vi "setUp.vi"(8 "error in (no error)":errorcluster, 11 "reference in":refnum<class "Import Export Test.lvclass">) -> (0 "error out":errorcluster, 3 "reference out":refnum<class "Import Export Test.lvclass">)   [LabVIEW 2019, in "Import Export Test.lvclass"]
doc: "setUp runs prior to the test method during test execution. Use this method to initialize any object data required by your tests."
uses:
  Import Export Test.lvclass
  C:/Program Files (x86)/National Instruments/LabVIEW 2019/vi.lib/addons/_JKI Toolkits/VI Tester/TestCase.llb/TestCase.lvclass
  NationalInstruments.VeriStand.SystemDefinitionAPI
  Import Export Test.lvclass/Import Export Test.ctl
  <userlib>/_OpenG.lib/file/file.llb/Append Path to Root if Relative - Scalar__ogtk.vi
  <vilib>/addons/_JKI Toolkits/VI Tester/TestCase.llb/TestCase.lvclass
  niveristand-custom-device-testing-tools/VeriStandTestUtilities/VeriStandTestUtilities.lvlib
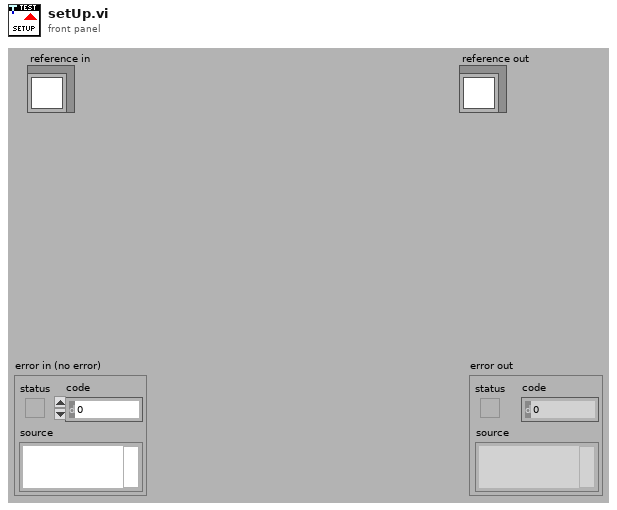
[diagram p1: front panel]
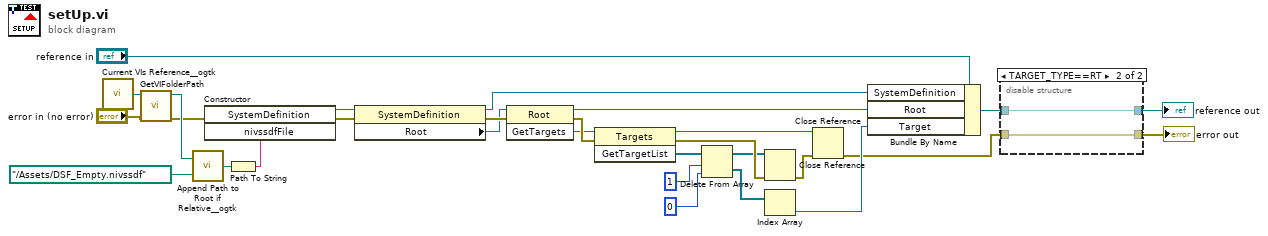
[diagram p0: block diagram]
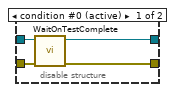
[diagram p2: hidden frame]
diagram:
  n1 = call <userlib>:"Current VIs Reference__ogtk.vi"() -> ("Current VI's reference"=w29:refnum<vi>)  [unwired: 5 in]
  n2 = call "GetVIFolderPath.vi"("error in (no error)"="error in (no error)", "VI Reference in"=w29) -> ("error out"=w25:errorcluster, "VI Folder Path out"=w28:path)  [unwired: 8 in]
  n3 = call-poly <userlib>:"Append Path to Root if Relative__ogtk.vi"("Absolute or Relative Path"=path "../Assets/DSF_Empty.nivssdf", "Root Path"=w28) -> ("Absolute or Appended Path"=w26:path)
  n4 = Path To String(path=w26) -> (string=w23:string)
  n5 = constructor class="SystemDefinition" ("Constructor Node")(error in=w25, "nivssdfFile"=w23) -> (reference out=w22:refnum<k24>, error out=w24:errorcluster)  [unwired: 2 in, 2 out]
  n6 = property on="Property Node" class="SystemDefinition"(reference=w22, error in=w24) -> (reference out=w7:refnum<k24>, error out=w21:errorcluster, "Root"=w20:refnum<k24>)
  n7 = invoke on="Invoke Node" class="Root" method="GetTargets"(reference=w20, error in=w21) -> (reference out=w8:refnum<k24>, error out=w19:errorcluster, "GetTargets"=w18:refnum<k24>)  [unwired: 1 in]
  n8 = invoke on="Invoke Node" class="Targets" method="GetTargetList"(reference=w18, error in=w19) -> (reference out=w11:refnum<k24>, error out=w14:errorcluster, "GetTargetList"=w17:refnum<k24>[])  [unwired: 1 in]
  n9 = Delete From Array(array=w17, length=1, index=0) -> (deleted portion=w10:refnum<k24>[], array with subset deleted=w13:refnum<k24>[])
  n10 = Close Reference(reference=w13, error in (no error)=w14) -> (error out=w12:errorcluster)
  n11 = Index Array(array=w10) -> (element=w9:refnum<k24>)  [unwired: 1 in]
  n12 = Close Reference(reference=w11, error in (no error)=w12) -> (error out=w5:errorcluster)
  n13 = Bundle By Name(cluster="reference in", "SystemDefinition"=w7, "Root"=w8, "Target"=w9) -> (w6:refnum<class "Import Export Test.lvclass">)
  n14 = disable-structure "Conditional Disable Structure" shown="TARGET_TYPE==RT" {
    disable-tunnel: w5 -> [w33 w34]
    disable-tunnel: [w32 w34] -> w2
    disable-tunnel: [w31 w35] -> w3
    disable-tunnel: w6 -> [w30 w35]
    frame condition #0 (active) {
      n15 = call <vilib>:"WaitOnTestComplete.vi"("error in (no error)"=w33, "TestCase in"=w30) -> ("error out"=w32:errorcluster, "TestCase out"=w31:refnum<class "Import Export Test.lvclass">)  [unwired: 8 in]
    }
    frame condition #1 {
    }
  }
  "error out" <- w2
  "reference out" <- w3
